vi "Test Set Row Values Bool.vi"(11 "Test Case In":refnum<class "Test Open Xml.lvclass">) -> (0 "error out":errorcluster, 3 "Test Case Out":refnum<class "Test Open Xml.lvclass">)   [LabVIEW 2025, in "Test Open Xml.lvclass"]
uses:
  Test Open Xml.lvclass
  C:/Program Files/National Instruments/LabVIEW 2025/vi.lib/Astemes/LUnit/Test Case.lvclass
  Source/Cell DataType.ctl
  <vilib>/Astemes/LUnit/Test Case.lvclass/Test Case.ctl
  <vilib>/Astemes/LUnit/Append Fail Result.vi
  <vilib>/Astemes/LUnit/Append Pass Result.vi
  <vilib>/Astemes/LUnit/Run In UI.vi
  <vilib>/Astemes/LUnit/Test Case.lvclass
  Source/Open Xml.lvlib
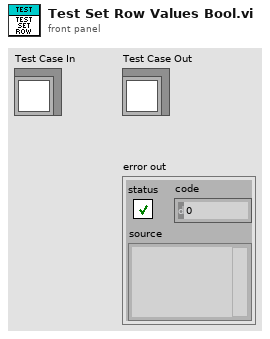
[diagram p1: front panel]
types:
  T1 = typedef "Open Xml.lvlib/Cell DataType.ctl" = enum16{"Void", "Boolean", "Number", "Error", "SharedString", "String", "InlineString", "Date"}
  T2 = cluster{"Number":dbl, "String":string, "Boolean":bool, "Time Stamp":timestamp, "Error":errorcluster}[]
  T3 = cluster{"Number":dbl, "String":string, "Boolean":bool, "Time Stamp":timestamp, "Error":errorcluster}
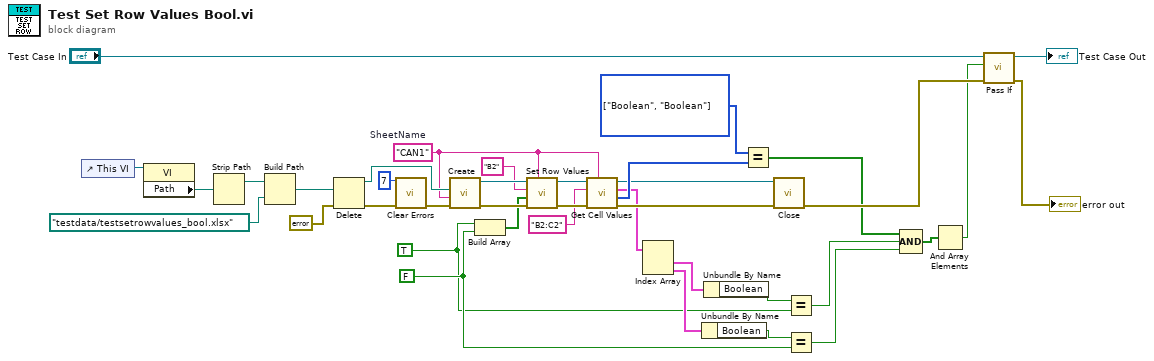
[diagram p0: block diagram]
diagram:
  w1 = TRUE
  w2 = FALSE
  w13 = T1[] [enum."Boolean", enum."Boolean"] items=["Void", "Boolean", "Number", "Error", "SharedString", "String", "InlineString", "Date"] ("x")
  w3 = "CAN1"  # SheetName
  n1 = control-ref of="This VI"() -> (w35:refnum<vi>)
  n2 = property class="VI"(reference=w35) -> ("Path"=w34:path)  [unwired: 1 in, 2 out]
  n3 = Strip Path(path=w34) -> (stripped path=w33:path)  [unwired: 1 out]
  n4 = Build Path(base path=w33, name or relative path=path "testdata/testsetrowvalues_bool.xlsx") -> (appended path=w23:path)
  n5 = Delete(path (use dialog)=w23, error in=errorcluster {"status"=FALSE, "code"=0, "source"=""}) -> (deleted path=w25:path, error out=w28:errorcluster)  [unwired: 3 in, 1 out]
  n6 = call <vilib>:"Clear Errors.vi"("error in (no error)"=w28, "specific error code to clear (0: all)"=7) -> ("error out"=w27:errorcluster)  [unwired: 4 in, 1 out]
  n7 = call "Create.vi"("error in"=w27, "SheetName"=w3, "Path"=w25) -> ("error out"=w30:errorcluster, "SpreadsheetDoc"=w31:refnum<k24>)  [unwired: 7 in]
  n8 = Build Array(w1, w2) -> (w8:bool[])
  n9 = call "Set Row Values.vi"("Sheet Name"=w3, "error in"=w30, "Values"=w8, "Cell Address"="B2", "SpreadsheetDoc"=w31) -> ("error out"=w20:errorcluster, "SpreadsheetDoc out"=w19:refnum<k24>)  [unwired: 5 in]
  n10 = call "Get Cell Values.vi"("Sheet Name"=w3, "error in"=w20, "Cell Addresses"="B2:C2" ("Cell Address"), "SpreadsheetDoc in"=w19) -> ("error out"=w22:errorcluster, "Types"=w18:T1[], "Cell Values"=w14:T2, "SpreadsheetDoc out"=w4:refnum<k24>)  [unwired: 4 in]
  n11 = Index Array(array=w14) -> (element #1=w12:T3, element #2=w11:T3)  [unwired: 2 in]
  n12 = Unbundle By Name(w11) -> ("Boolean"=w6:bool)
  n13 = Unbundle By Name(w12) -> ("Boolean"=w9:bool)
  n14 = Equal?(x=w13, y=w18) -> (x = y?=w17:bool[])
  n15 = call "Close.vi"("error in"=w22, "SpreadsheetDoc"=w4) -> ("error out"=w24:errorcluster)  [unwired: 9 in]
  n16 = Equal?(x=w9, y=w1) -> (x = y?=w5:bool)
  n17 = Equal?(x=w6, y=w2) -> (x = y?=w7:bool)
  n18 = Compound Arithmetic op=AND(w17, w5, w7) -> (w10:bool[])
  n19 = And Array Elements(Boolean array=w10) -> (logical AND=w21:bool)
  n20 = call <vilib>:"Pass If.vi"("error in (no error)"=w24, "Pass?"=w21, "LUnit Test Case In"="Test Case In") -> ("error out"=→"error out":errorcluster, "LUnit Test Case Out"=→"Test Case Out":refnum<class "Test Open Xml.lvclass">)  [unwired: 7 in]
